vi "PrintAllDevices.vi"(7 "Path":path=path "C:/LabViewTesty", 9 "Colors 5":u32[](array[colorbox])=[11796480, 37103, 40712, 16770816, 11796658, 4210752, 9567230, 16741120, 750336, 786687, 7565056, 16777222, 11121611, 2817859, 16728723, 16711686, 4340736], 10 "Dev":i32[](array[numeric]), 11 "All pacets devices":picture) -> ()   [LabVIEW 2014]
panel:
  out "Packets and Devices":T1={"All pacets devices"=bytes[270], "Colors 5"=[11796480, 37103, 40712, 16770816, 11796658, 4210752, 9567230, 16741120, 750336, 786687, 7565056, 16777222, 11121611, 2817859, 16728723, 16711686, 4340736], "Data"="", "Time"="", "Dev"=[]}
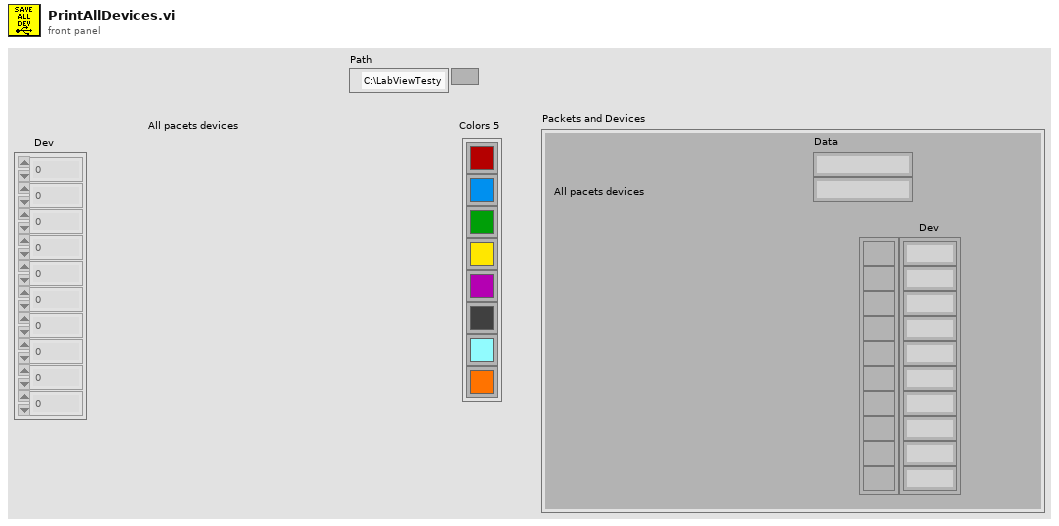
[diagram p1: front panel]
types:
  T1 = cluster{"All pacets devices":picture, "Colors 5":u32[], "Data":string, "Time":string, "Dev":i32[]}
  T2 = typedef "imagedata.ctl" = cluster{"image type":i32, "image depth":i32, "image":u8[], "mask":u8[], "colors":u32[], "Rectangle":cluster{"left":i16, "top":i16, "right":i16, "bottom":i16}}
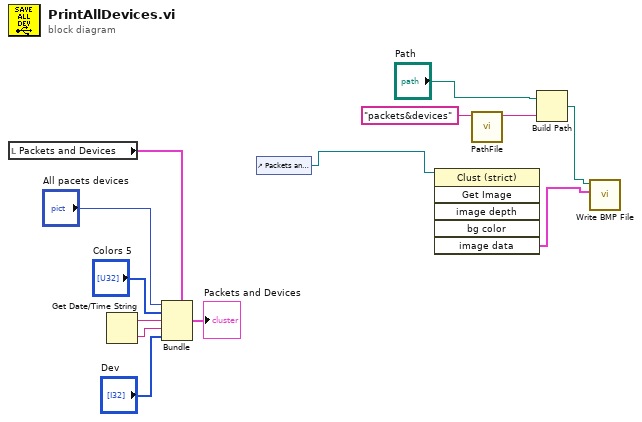
[diagram p0: block diagram]
diagram:
  n1 = local read "Packets and Devices"() -> (w13:T1)
  n2 = Get Date/Time String() -> (date string=w11:string, time string=w10:string)  [unwired: 3 in]
  n3 = Bundle(cluster=w13, "All pacets devices"="All pacets devices", "Colors 5"="Colors 5", "Data"=w11, "Time"=w10, "Dev"="Dev") -> (→"Packets and Devices":T1)
  n4 = control-ref of="Packets and Devices"() -> (w1:refnum<vi>)
  n5 = invoke class="Clust (strict)" method="Get Image"(reference=w1) -> ("image data"=w6:T2)  [unwired: 5 in, 5 out]
  n6 = call "PathFile.vi"("NameFile"="packets&devices") -> ("stringNameFile"=w2:string)  [unwired: 10 in]
  n7 = Build Path(base path="Path", name or relative path=w2) -> (appended path=w5:path)
  n8 = call <vilib>:"Write BMP File.vi"("image data"=w6, "path to BMP file"=w5) -> ()  [unwired: 8 in, 2 out]
